vi "ROS_Master_WebPageServer.vi"(5 "occurrence":refnum<k4>) -> ()   [LabVIEW 2012]
uses:
  <userlib>/ROSforLV/ROS/Code/_ROSDefinition.vi
panel:
  out "requests":string[](array[string])
  out "Last Reply":string="HTTP/1.1 200 OK\r\nUser-Agent: LabVIEW WebServer/0.1\nDate: Thu, 08 Dec 2011 18:58:48 GMT\nExpires: Thu, 08 Dec 2011 18:58:48 GMT\nIgnore-Buffer: xXxBUFFERxXx\nContent-Type: text/html\nContent-Length: 508\nConnection: keep-alive\r\n\r\n<!DOCTYPE HTML PUBLIC \"-//W3C//DTD HTML 4.0 Transitional//EN\">\n<HTML>\n<!-- Constructed with LabVIEW Report Generation -->\n<HEAD>\n<TITLE></TITLE>\n</HEAD>\n\n<BODY>\n\n<form name=\"myform\" action=\"index.htm\" method=\"POST\">\n\n<br><br>\n____<input type=\"submit\" name=\"1\" value=\"forward\"> \n<br><br>\n<input type=\"submit\" name=\"2\" value=\"left\"> \n<input type=\"submit\" name=\"0\" value=\"STOP\"> \n<input type=\"submit\" name=\"3\" value=\"right\">\n<br><br>\n_____<input type=\"submit\" name=\"4\" value=\"back\"> \n\n</form>\n\n</BODY>\n\n</HTML>\r\n\r\n"
  in  "stop":bool
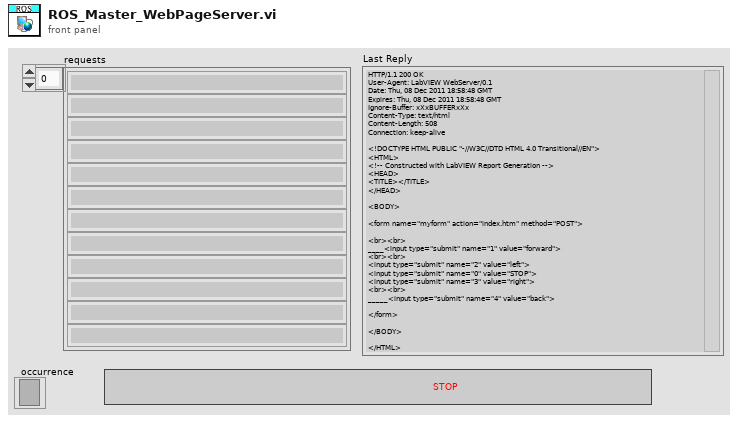
[diagram p1: front panel]
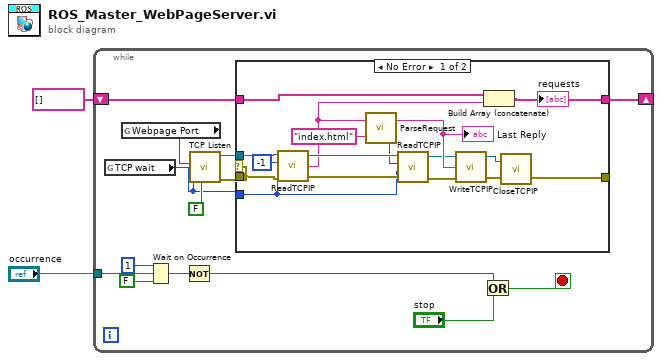
[diagram p0: block diagram]
diagram:
  n1 = while {
    shift-right: [w11] -> _
    shift-left: string[] [] -> [w10]
    tunnel: "occurrence" -> [w9]
    stop <- w4 stop-if-true
    n2 = global read "_ROSDefinition.vi" "TCP wait"() -> (w13:i32)
    n3 = global read "_ROSDefinition.vi" "Webpage Port"() -> (w12:u16)
    n4 = Wait on Occurrence(1:FALSE ("ignore previous (T)"), 2:w9, 3:1 ("ms timeout (-1)")) -> (0:w6:bool)
    n5 = Not(x=w6) -> (.not. x?=w3:bool)
    n6 = call <vilib>:"TCP Listen.vi"("resolve remote address (T)"=FALSE, "timeout ms (wait forever: -1)"=w13, "port"=w12) -> ("error out"=w15:errorcluster, "connection ID"=w14:refnum<k5>)  [unwired: 4 in, 3 out]
    n7 = case shown="No Error" w15 {
      tunnel: w14 -> [w33 _]
      tunnel: w15 -> [w30 _]
      tunnel: [w23 _] -> _
      tunnel: w13 -> [w21 _]
      tunnel: [w18 w34] -> w11
      tunnel: w10 -> [w17 w34]
      frame No Error {
        n8 = call <userlib>:"ReadTCPIP.vi"("error in"=w30, "TCP Timeout"=w21, "bytes to read"=-1, "connection ID"=w33) -> ("errorout"=w26:errorcluster, "String"=w19:string, "connection ID Out"=w28:refnum<k5>)
        n9 = call <userlib>:"ParseRequest.vi"("Node html"="index.html", "String in"=w19) -> ("Post size"=w27:i32, "Reply"=w29:string)
        "Last Reply" <- w29
        n10 = call <userlib>:"ReadTCPIP.vi"("error in"=w26, "TCP Timeout"=w21, "bytes to read"=w27, "connection ID"=w28) -> ("errorout"=w25:errorcluster, "connection ID Out"=w24:refnum<k5>)  [unwired: 1 out]
        n11 = call <userlib>:"WriteTCPIP.vi"("error in"=w25, "String"=w29, "connection ID"=w24) -> ("errorout"=w32:errorcluster, "connection ID Out"=w31:refnum<k5>)  [unwired: 1 in]
        n12 = Build Array (concatenate)(w17, w19) -> (w18:string[])
        "requests" <- w18
        n13 = call <userlib>:"CloseTCPIP.vi"("error in (no error)"=w32, "connection ID"=w31) -> ("error out"=w23:errorcluster)  [unwired: 1 in]
      }
      frame Error {
      }
    }
    n14 = Or(x=w3, y="stop") -> (x .or. y?=w4:bool)
  }
